vi "Servo Pulse Gen..vi"() -> ()   [LabVIEW 2015]
uses:
  Slide Servo.ctl
  Galobal variable_TI.vi
  Project Setup/Globle Variable/GR_Servo.vi
panel:
  out "Enum":T1
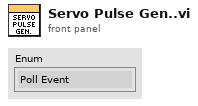
[diagram p1: front panel]
types:
  T1 = typedef "Slide Servo.ctl" = enum16{"Poll Event", "Servo CMD", "Slide Servo Home ", "Exit"}
  T2 = cluster{"Emergency_1":bool, "Reset_2":bool, "Air Pressure_4":bool, "Safety Sensor_5":bool, "Safety Sensor_6":bool, "Barcode Rev rs_24":bool, "Clamp fwd rs_21":bool, "Servo Fault":bool, "Home _3":bool}
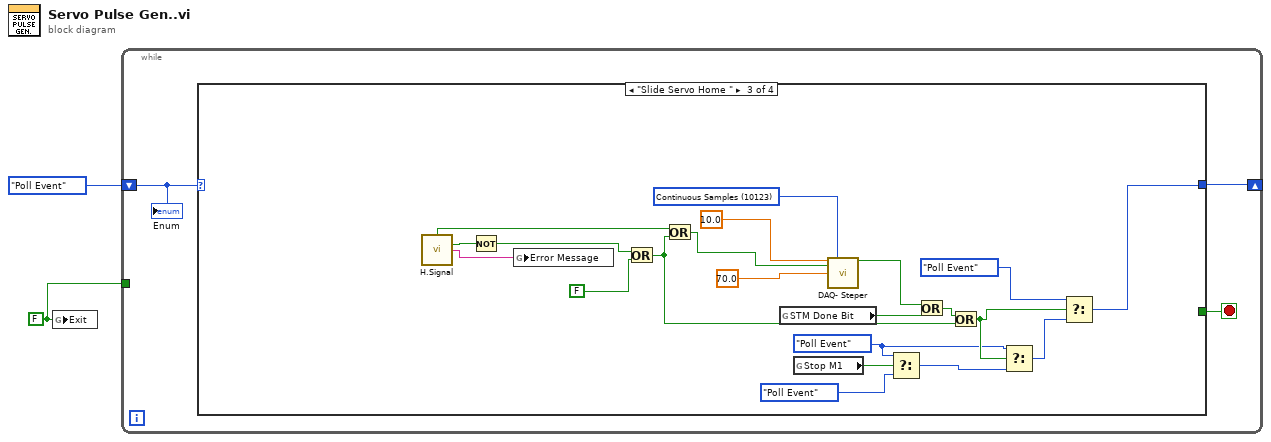
[diagram p0: block diagram]
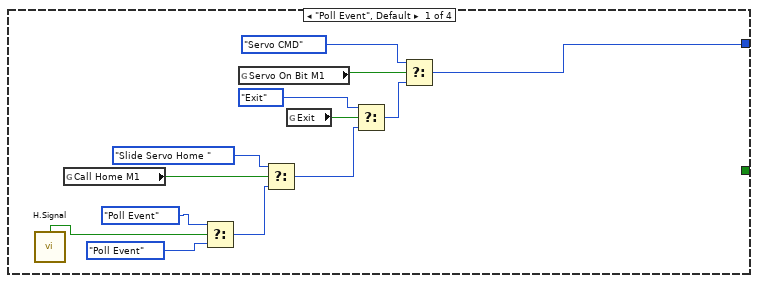
[diagram p2: hidden frame]
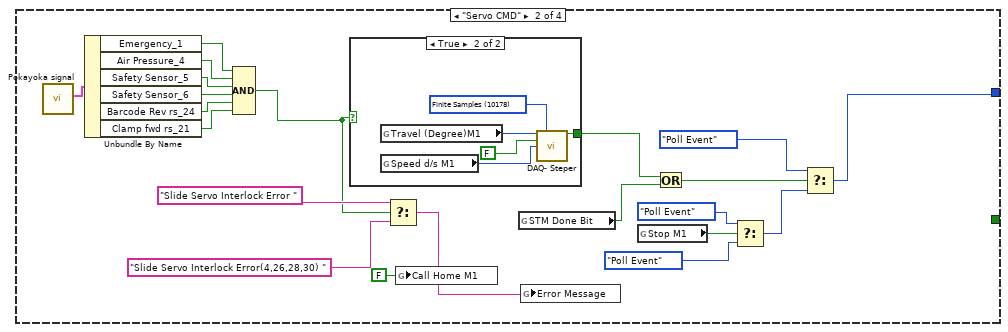
[diagram p3: hidden frame]
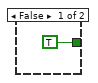
[diagram p4: hidden frame]
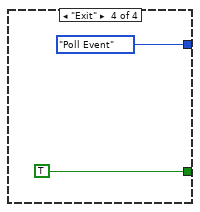
[diagram p5: hidden frame]
diagram:
  w1 = FALSE ("Exit")
  n1 = global write "Galobal variable_TI.vi" "Exit"(w1) -> ()
  n2 = while {
    shift-right: [w4] -> _
    shift-left: Slide_Servo."Poll Event" ("Enum") -> [w5]
    tunnel: w1 -> [_]
    stop <- w3 stop-if-true
    n3 = case shown="\"Slide Servo Home \"" w5 {
      tunnel: [w13 w35 w55 Slide_Servo."Poll Event" ("Enum")] -> w4
      tunnel: [_ _ _ TRUE] -> w3
      frame "Poll Event", Default {
        n4 = call "H.Signal.vi"() -> ("element"=w6:bool)  [unwired: 10 in, 5 out]
        n5 = global read "Galobal variable_TI.vi" "Call Home M1"() -> (w11:bool)
        n6 = Select(t=Slide_Servo."Poll Event" ("Enum"), s=w6, f=Slide_Servo."Poll Event" ("Enum")) -> (s? t:f=w8:T1)
        n7 = global read "GR_Servo.vi" "Servo On Bit M1"() -> (w16:bool)
        n8 = Select(t=Slide_Servo."Slide Servo Home " ("Enum"), s=w11, f=w8) -> (s? t:f=w10:T1)
        n9 = global read "Galobal variable_TI.vi" "Exit"() -> (w17:bool)
        n10 = Select(t=Slide_Servo."Exit" ("Enum"), s=w17, f=w10) -> (s? t:f=w18:T1)
        n11 = Select(t=Slide_Servo."Servo CMD" ("Enum"), s=w16, f=w18) -> (s? t:f=w13:T1)
      }
      frame "Servo CMD" {
        n12 = call "Pokayoka signal.vi"() -> ("output cluster"=w26:T2)  [unwired: 10 in, 1 out]
        n13 = Unbundle By Name(w26) -> ("Emergency_1"=w19:bool, "Air Pressure_4"=w25:bool, "Safety Sensor_5"=w24:bool, "Safety Sensor_6"=w23:bool, "Barcode Rev rs_24"=w22:bool, "Clamp fwd rs_21"=w21:bool)
        n14 = Compound Arithmetic op=AND(w19, w25, w24, w23, w22, w21) -> (w20:bool)
        n15 = case shown="True" w20 {
          tunnel: [TRUE ("Task Done Bit") w43] -> w39
          frame False {
          }
          frame True {
            w41 = 10178 items=["Finite Samples"=10178, "Continuous Samples"=10123, "Hardware Timed Single Point"=12522] ("Mode")
            n16 = global read "GR_Servo.vi" "Travel (Degree)M1"() -> (w44:i32)
            n17 = global read "GR_Servo.vi" "Speed d/s M1"() -> (w45:i32)
            n18 = call "DAQ- Steper.vi"("Travel (Degree)"=w44, "Mode"=w41, "Home Condition"=FALSE, "Speed d/s"=w45) -> ("Task Done Bit"=w43:bool)  [unwired: 10 in, 1 out]
          }
        }
        n19 = Select(t="Slide Servo Interlock Error ", s=w20, f="Slide Servo Interlock Error(4,26,28,30) ") -> (s? t:f=w27:string)
        n20 = global write "Galobal variable_TI.vi" "Call Home M1"(FALSE ("Call Home M1")) -> ()
        n21 = global read "Galobal variable_TI.vi" "STM Done Bit"() -> (w38:bool)
        n22 = global write "GR_Servo.vi" "Error Message"(w27) -> ()
        n23 = global read "Galobal variable_TI.vi" "Stop M1"() -> (w34:bool)
        n24 = Or(x=w39, y=w38) -> (x .or. y?=w37:bool)
        n25 = Select(t=Slide_Servo."Poll Event" ("Enum"), s=w34, f=Slide_Servo."Poll Event" ("Enum")) -> (s? t:f=w31:T1)
        n26 = Select(t=Slide_Servo."Poll Event" ("Enum"), s=w37, f=w31) -> (s? t:f=w35:T1)
      }
      frame "Slide Servo Home " {
        w54 = 10123 items=["Finite Samples"=10178, "Continuous Samples"=10123, "Hardware Timed Single Point"=12522] ("Mode")
        w57 = Slide_Servo."Poll Event" ("Enum")
        n27 = call "H.Signal.vi"() -> ("element"=w47:bool, "HI Bit Auto"=w50:bool, "Error M Auto"=w51:string)  [unwired: 10 in, 3 out]
        n28 = Not(x=w50) -> (.not. x?=w49:bool)
        n29 = global write "GR_Servo.vi" "Error Message"(w51) -> ()
        n30 = Or(x=w49, y=FALSE) -> (x .or. y?=w48:bool)
        n31 = Or(x=w47, y=w48) -> (x .or. y?=w46:bool)
        n32 = global read "Galobal variable_TI.vi" "STM Done Bit"() -> (w65:bool)
        n33 = global read "Galobal variable_TI.vi" "Stop M1"() -> (w61:bool)
        n34 = call "DAQ- Steper.vi"("Travel (Degree)"=10.0, "Mode"=w54, "Home Condition"=w46, "Speed d/s"=70.0) -> ("Task Done Bit"=w66:bool)  [unwired: 10 in, 1 out]
        n35 = Select(t=w57, s=w61, f=Slide_Servo."Poll Event" ("Enum")) -> (s? t:f=w58:T1)
        n36 = Or(x=w66, y=w65) -> (x .or. y?=w62:bool)
        n37 = Or(x=w62, y=w48) -> (x .or. y?=w59:bool)
        n38 = Select(t=w57, s=w59, f=w58) -> (s? t:f=w56:T1)
        n39 = Select(t=Slide_Servo."Poll Event" ("Enum"), s=w59, f=w56) -> (s? t:f=w55:T1)
      }
      frame "Exit" {
      }
    }
    "Enum" <- w5
  }
